vi "json_parse_key.vi"(8 "error in (no error)":errorcluster, 9 "offset (0)":i32, 11 "data":string) -> (0 "error out":errorcluster, 1 "offset past match":i32, 2 "key":string)   [LabVIEW 2017]
uses:
  <vilib>/regexp/Match Regular Expression.xnode
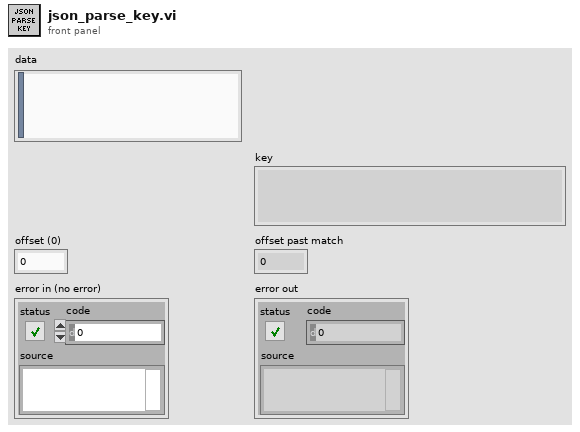
[diagram p1: front panel]
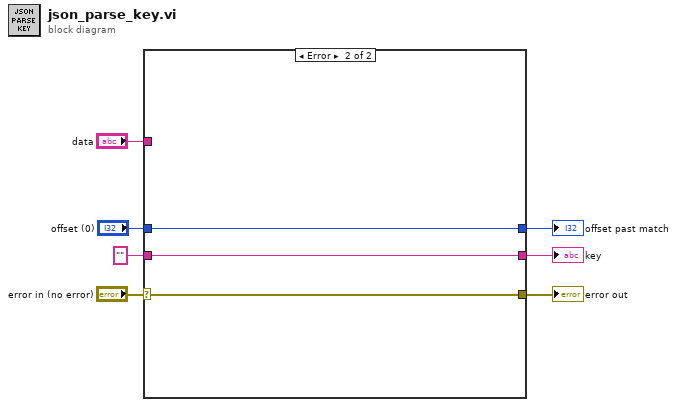
[diagram p0: block diagram]
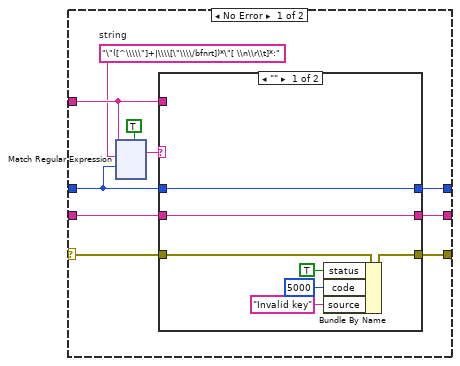
[diagram p2: hidden frame]
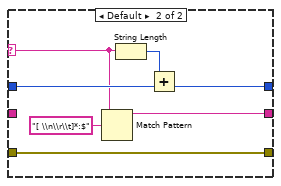
[diagram p3: hidden frame]
diagram:
  n1 = case shown="Error" "error in (no error)" {
    selector: "error in (no error)" -> [w16 w148]
    tunnel: [w17 w148] -> w7
    tunnel: [w15 w147] -> w5
    tunnel: "data" -> [w14 _]
    tunnel: "" -> [w13 w147]
    tunnel: "offset (0)" -> [w11 w146]
    tunnel: [w12 w146] -> w1
    frame No Error {
      w10 = "\"([^\\\\\"]+|\\\\[\"\\\\/bfnrt])*\"[ \\n\\r\\t]*:"  # string
      n2 = xnode "Match Regular Expression"("input string"=w14, "regular expression"=w10, "offset (0)"=w11, "multiline? (F)"=TRUE) -> ("whole match"=w8:string)  [unwired: 2 in, 4 out]
      n3 = case shown="\"\"" w8 {
        selector: w8 -> [_ w26]
        tunnel: w14 -> [_ _]
        tunnel: [w23 w31] -> w17
        tunnel: w16 -> [w24 w31]
        tunnel: [w19 w28] -> w15
        tunnel: w13 -> [w19 _]
        tunnel: w11 -> [w18 w30]
        tunnel: [w18 w29] -> w12
        frame "" {
          n4 = Bundle By Name(cluster=w24, "status"=TRUE, "code"=5000, "source"="Invalid key") -> (w23:errorcluster)
        }
        frame Default {
          n5 = Match Pattern(string=w26, regular expression="[ \\n\\r\\t]*:$") -> (before substring=w28:string)  [unwired: 1 in, 3 out]
          n6 = String Length(string=w26) -> (length=w25:i32)
          n7 = Add(x=w25, y=w30) -> (x+y=w29:i32)
        }
      }
    }
    frame Error {
    }
  }
  "error out" <- w7
  "key" <- w5
  "offset past match" <- w1
